vi "GETENUMdll_Test.vi"(8 "error in (no error)":errorcluster) -> (0 "error out":errorcluster, 3 "Passed?":bool)   [LabVIEW 2016]
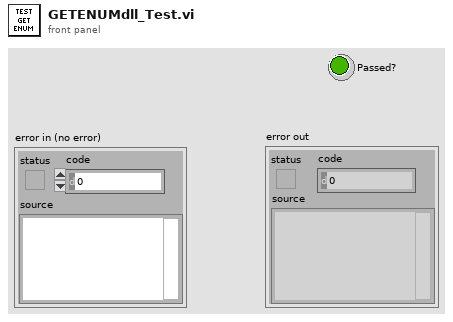
[diagram p1: front panel]
types:
  T1 = cluster{"iEnum":i32, "ierr":i32, "herr":string, "hEnum_length":i32, "herr_length":i32}
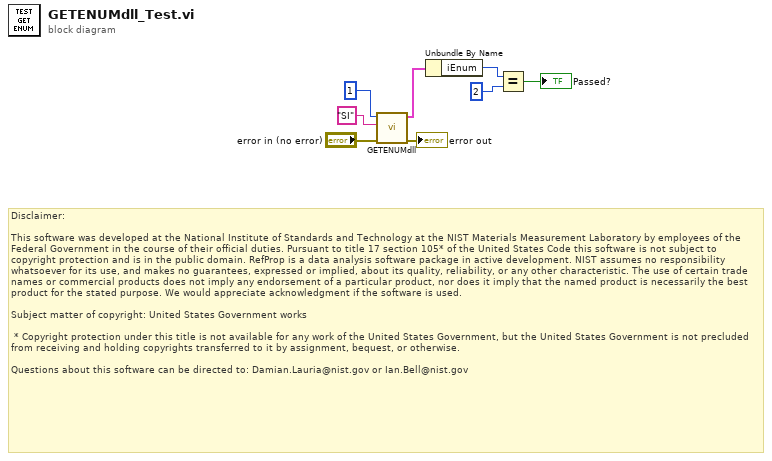
[diagram p0: block diagram]
diagram:
  # "Disclaimer:\n\nThis software was developed at the National Institute of Standards and Technology at the NIST Materials Measurement Laboratory by employees of the Federal Government in the course of their official duties. Pursuant to title 17 section 105* of the United States Code this software is not subject to copyright protection and is in the public domain. RefProp is a data analysis software package in active development. NIST assumes no responsibility whatsoever for its use, and makes no guarantees, expressed or implied, about its quality, reliability, or any other characteristic. The use of certain trade names or commercial products does not imply any endorsement of a particular product, nor does it imply that the named product is necessarily the best product for the stated purpose. We would appreciate acknowledgment if the software is used.\n \nSubject matter of copyright: United States Government works\n  \n * Copyright protection under this title is not available for any work of the United States Government, but the United States Government is not precluded from receiving and holding copyrights transferred to it by assignment, bequest, or otherwise.\n\nQuestions about this software can be directed to: Damian.Lauria@nist.gov or Ian.Bell@nist.gov"
  n1 = call "GETENUMdll.vi"("error in (no error)"="error in (no error)", "hEnum"="SI", "iFlag"=1) -> ("error out"=→"error out":errorcluster, "Outputs"=w4:T1)  [unwired: 7 in]
  n2 = Unbundle By Name(w4) -> ("iEnum"=w3:i32)
  n3 = Equal?(x=w3, y=2) -> (x = y?=→"Passed?":bool)
